vi "vipb_prebuild_Execute Unit Tests.vi"(10 "Variant":variant) -> (0 "error out":errorcluster)   [LabVIEW 2013]
uses:
  <vilib>/addons/_JKI Toolkits/VI Tester/TestSuite.llb/TestSuite.lvclass
  <vilib>/addons/_JKI Toolkits/VI Tester/VI Tester API.llb/Run Tests (Test Object).vi
  <vilib>/addons/_JKI Toolkits/VI Tester/VI Tester API.llb/VI Tester API.lvlib
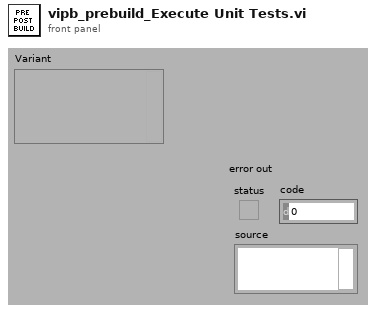
[diagram p1: front panel]
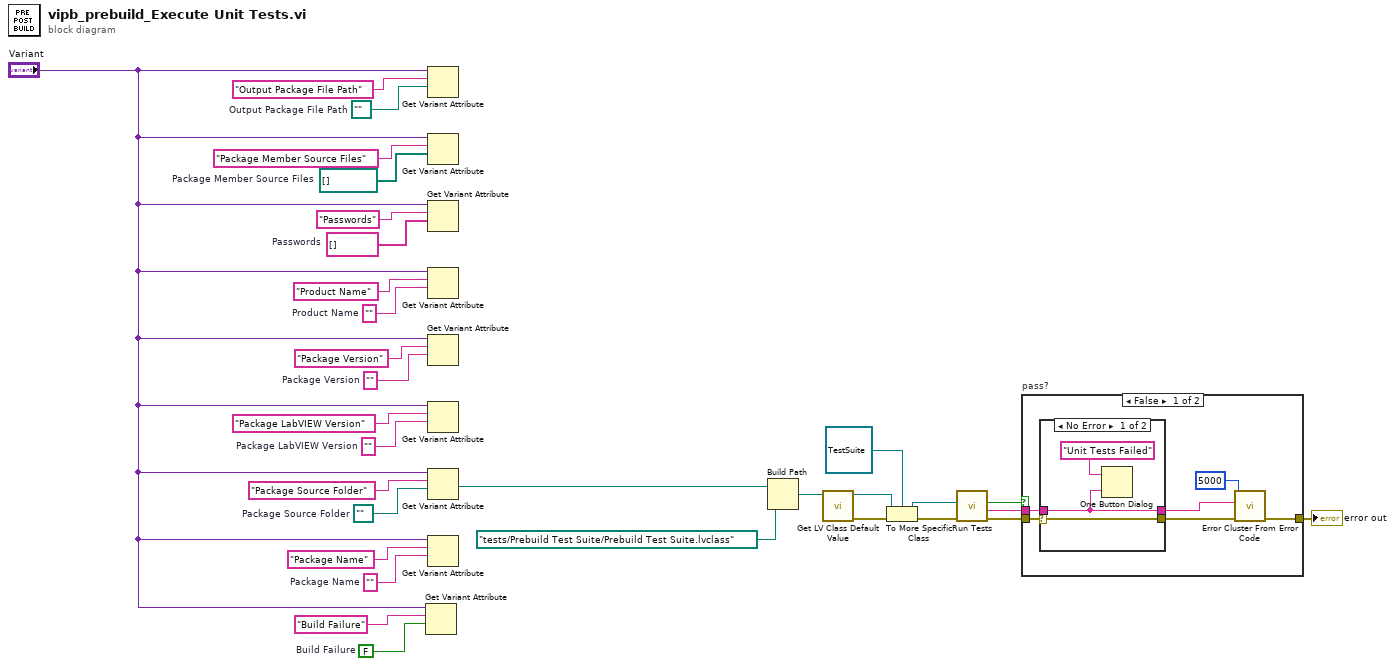
[diagram p0: block diagram]
diagram:
  w14 = FALSE  # Build Failure
  w16 = path ""  # Package Source Folder
  w17 = ""  # Package Name
  w20 = ""  # Package LabVIEW Version
  w22 = ""  # Package Version
  w24 = ""  # Product Name
  w26 = string[] []  # Passwords
  w28 = path[] []  # Package Member Source Files
  w30 = path ""  # Output Package File Path
  n1 = Get Variant Attribute(Variant="Variant", name="Build Failure", default value (empty Variant)=w14) -> ()  [unwired: 1 in, 4 out]
  n2 = Get Variant Attribute(Variant="Variant", name="Output Package File Path", default value (empty Variant)=w30) -> ()  [unwired: 1 in, 4 out]
  n3 = Get Variant Attribute(Variant="Variant", name="Package Member Source Files", default value (empty Variant)=w28) -> ()  [unwired: 1 in, 4 out]
  n4 = Get Variant Attribute(Variant="Variant", name="Passwords", default value (empty Variant)=w26) -> ()  [unwired: 1 in, 4 out]
  n5 = Get Variant Attribute(Variant="Variant", name="Product Name", default value (empty Variant)=w24) -> ()  [unwired: 1 in, 4 out]
  n6 = Get Variant Attribute(Variant="Variant", name="Package Version", default value (empty Variant)=w22) -> ()  [unwired: 1 in, 4 out]
  n7 = Get Variant Attribute(Variant="Variant", name="Package LabVIEW Version", default value (empty Variant)=w20) -> ()  [unwired: 1 in, 4 out]
  n8 = Get Variant Attribute(Variant="Variant", name="Package Source Folder", default value (empty Variant)=w16) -> (value=w2:path)  [unwired: 1 in, 3 out]
  n9 = Get Variant Attribute(Variant="Variant", name="Package Name", default value (empty Variant)=w17) -> ()  [unwired: 1 in, 4 out]
  n10 = Build Path(base path=w2, name or relative path=path "tests/Prebuild Test Suite/Prebuild Test Suite.lvclass") -> (appended path=w10:path)
  n11 = call <vilib>:"Get LV Class Default Value.vi"("class path"=w10) -> ("error out"=w7:errorcluster, "object"=w5:refnum<class>)  [unwired: 9 in]
  n12 = To More Specific Class(target class=refnum<class "TestSuite.lvclass"> refnum ("TestSuite.lvclass"), reference=w5, error in=w7) -> (specific class reference=w3:refnum<class "TestSuite.lvclass">, error out=w6:errorcluster)
  n13 = call-poly <vilib>:"Run Tests.vi"("error in (no error)"=w6, "Test"=w3) -> ("error out"=w12:errorcluster, "test details"=w8:string, "successful?"=w9:bool)  [unwired: 7 in]
  n14 = case "pass?" shown="False" w9 {
    tunnel: [w36 w43] -> w1
    tunnel: w12 -> [w34 w43]
    tunnel: w8 -> [w35 _]
    frame False {
      n15 = case shown="No Error" w34 {
        selector: w34 -> [w39 w42]
        tunnel: w35 -> [w38 w41]
        tunnel: [w39 w42] -> w33
        tunnel: [w38 w41] -> w32
        frame No Error {
          n16 = One Button Dialog(message="Unit Tests Failed" ("title"), button name ("OK")=w38) -> ()  [unwired: 1 out]
        }
        frame Error {
        }
      }
      n17 = call <vilib>:"Error Cluster From Error Code.vi"("error in (no error)"=w33, "error message (\"\")"=w32, "error code (0)"=5000) -> ("error out"=w36:errorcluster)  [unwired: 6 in]
    }
    frame True {
    }
  }
  "error out" <- w1
